vi "GetFlowmeterData.vi"(6 "Graph in":cluster{dbl[], dbl[]}, 7 "Index":i32=250, 8 "error in":errorcluster, 9 "Length":i32=250, 11 "ON":bool) -> (0 "error out":errorcluster, 2 "Values":cluster{dbl[], dbl[]})   [LabVIEW 2012]
uses:
  GlobalVariables/HardwarePresent.vi
  GlobalVariables/CalibrationState.vi
  GlobalVariables/Samples.vi
  GlobalVariables/CurrentFlow.vi
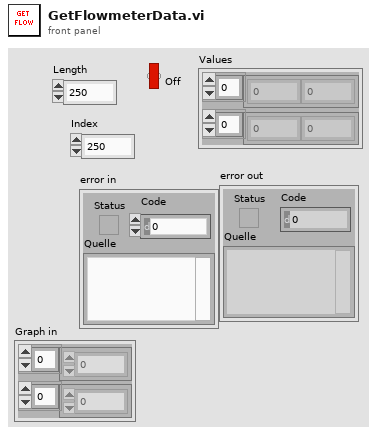
[diagram p1: front panel]
types:
  T1 = cluster{"CalibrationDone":bool, "CalibrationStep":u32, "Constante":dbl[], "Gain":dbl[]}
  T2 = cluster{"Pressure":cluster{"TimeSamples":dbl[], "PressureSamples":dbl[]}, "Flow":cluster{"TimeSamples":dbl[], "FlowSamples":dbl[]}}
  T3 = cluster{"TimeSamples":dbl[], "PressureSamples":dbl[]}
  T4 = cluster{"Pressure":cluster{"TimeSamples":dbl[], "PressureSamples":dbl[]}, cluster{dbl[], dbl[]}}
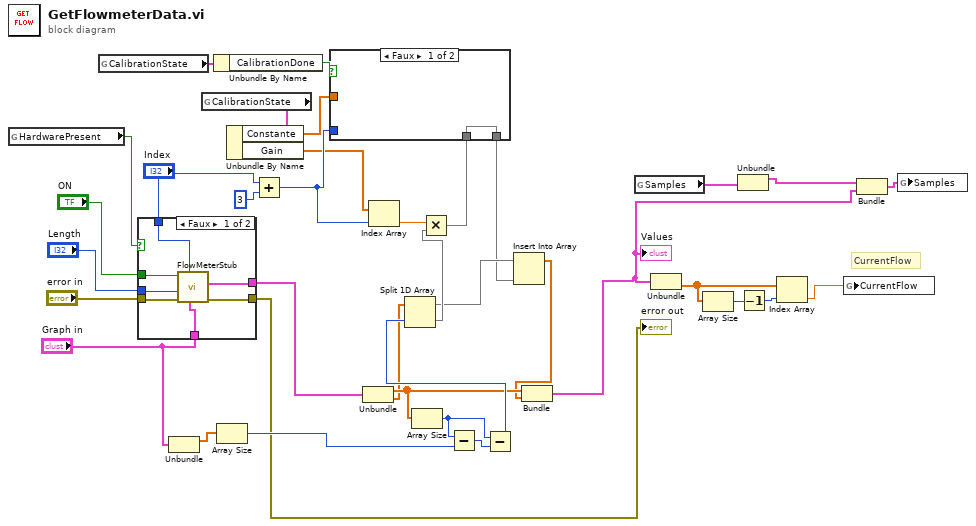
[diagram p0: block diagram]
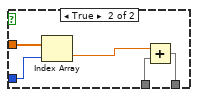
[diagram p2: hidden frame]
diagram:
  # "CurrentFlow"
  n1 = global read "HardwarePresent.vi" "HardwarePresent"() -> (w30:bool)
  n2 = global read "CalibrationState.vi" "CalibrationState"() -> (w28:T1)
  n3 = case shown="Faux" w30 {
    tunnel: "Graph in" -> [w40 w44]
    tunnel: "error in" -> [w39 w45]
    tunnel: [w41 w45] -> w1
    tunnel: [w42 w44] -> w8
    tunnel: "Length" -> [w38 _]
    tunnel: "ON" -> [w37 _]
    tunnel: "Index" -> [w43 _]
    frame False {
      n4 = call "FlowMeterStub.vi"("Graph in"=w40, "Index"=w43, "error in"=w39, "Length"=w38, "ON"=w37) -> ("error out"=w41:errorcluster, "Values"=w42:cluster{dbl[], dbl[]})  [unwired: 5 in]
    }
    frame True {
    }
  }
  "error out" <- w1
  n5 = Unbundle("Graph in") -> (w21:dbl[])  [unwired: 1 out]
  n6 = global read "CalibrationState.vi" "CalibrationState"() -> (w19:T1)
  n7 = Unbundle By Name(w28) -> ("CalibrationDone"=w27:bool)
  n8 = Array Size(array=w21) -> (size(s)=w7:i32)
  n9 = Unbundle By Name(w19) -> ("Constante"=w9:dbl[], "Gain"=w4:dbl[])
  n10 = Add(x="Index", y=3) -> (x+y=w5:i32)
  n11 = Unbundle(w8) -> (w13:dbl[], w12:dbl[])
  n12 = Index Array(array=w4, index=w5) -> (element=w16:dbl)
  n13 = Array Size(array=w13) -> (size(s)=w18:i32)
  n14 = Subtract(x=w18, y=w7) -> (x-y=w14:i32)
  n15 = Subtract(x=w18, y=w14) -> (x-y=w15:i32)
  n16 = Split 1D Array(array=w12, index=w15) -> (first subarray=w10:dbl[], second subarray=w17:dbl[])
  n17 = Multiply(x=w16, y=w17) -> (x*y=w3:dbl[])
  n18 = case shown="Faux" w27 {
    tunnel: w5 -> [_ w50]
    tunnel: w9 -> [_ w49]
    tunnel: w3 -> [w46 w48]
    tunnel: [w46 w47] -> w2
    frame False {
    }
    frame True {
      n19 = Index Array(array=w49, index=w50) -> (element=w51:dbl)
      n20 = Add(x=w51, y=w48) -> (x+y=w47:dbl[])
    }
  }
  n21 = Insert Into Array(array=w10, new element=w2) -> (w11:dbl[])  [unwired: 1 in]
  n22 = Bundle(w13, w11) -> (w6:cluster{dbl[], dbl[]})  [unwired: 1 in]
  "Values" <- w6
  n23 = global read "Samples.vi" "Samples"() -> (w24:T2)
  n24 = Unbundle(w6) -> (w36:dbl[])  [unwired: 1 out]
  n25 = Array Size(array=w36) -> (size(s)=w35:i32)
  n26 = Unbundle(w24) -> ("Pressure"=w22:T3)  [unwired: 1 out]
  n27 = Decrement(x=w35) -> (x-1=w34:i32)
  n28 = Index Array(array=w36, index=w34) -> (element=w29:dbl)
  n29 = global write "CurrentFlow.vi" "CurrentFlow"(w29) -> ()
  n30 = Bundle("Pressure"=w22, w6) -> (w23:T4)  [unwired: 1 in]
  n31 = global write "Samples.vi" "Samples"(w23) -> ()
